vi "niDAQmx Timing (Implicit).vi"(0 "task in":refnum<class "Session Factory.lvclass">, 1 "samples per channel":i32=1000, 2 "sample mode":i32(ring)=10178 items=["Finite Samples"=10178, "Continuous Samples"=10123, "Hardware Timed Single Point"=12522], 11 "error in":errorcluster) -> (4 "task out":refnum<class "Session Factory.lvclass">, 15 "error out":errorcluster)   [LabVIEW 2021, in "Session Management niDAQmx.lvlib" / "Session Factory.lvclass"]
doc: "Sets only the number of samples to acquire or generate without specifying timing. Typically, you should use this instance when the task does not require sample timing, such as tasks that use counters for buffered frequency measurement, buffered period measurement, or pulse train generation. For finite counter output tasks, <B>samples per channel</B> is the number of pulses to generate."
uses:
  Session Factory.lvclass
  NI_DAQmx_client/RPC Messages/nidaqmx_grpc_CfgImplicitTimingRequest.ctl
  NI_DAQmx_client/RPC Messages/nidevice_grpc_Session.ctl
  NI_DAQmx_client/RPC Messages/nidevice_grpc_Session_session/nidevice_grpc_Session_session.lvclass
  NI_DAQmx_client/RPC Messages/nidaqmx_grpc_CfgImplicitTimingRequest_sample_mode_enum/nidaqmx_grpc_CfgImplicitTimingRequest_sample_mode_enum.lvclass
  Session Factory.lvclass/Session Factory.ctl
  NI_DAQmx_client/RPC Messages/nidaqmx_grpc_AcquisitionType.ctl
  NI_DAQmx_client/RPC Messages/nidaqmx_grpc_CfgImplicitTimingRequest_sample_mode_enum/nidaqmx_grpc_CfgImplicitTimingRequest_sample_mode_enum.lvclass/nidaqmx_grpc_CfgImplicitTimingRequest_sample_mode_enum.ctl
  NI_DAQmx_client/NI_DAQmx_client.lvlib
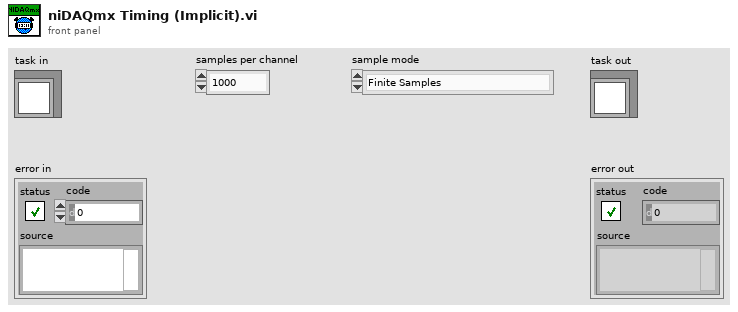
[diagram p1: front panel]
types:
  T1 = typedef "NI_DAQmx_client.lvlib/nidaqmx_grpc_CfgImplicitTimingRequest.ctl" = cluster{"task":T2, "nidaqmx_grpc_CfgImplicitTimingRequest_sample_mode_enum":refnum<class "nidaqmx_grpc_CfgImplicitTimingRequest_sample_mode_enum.lvclass">, "samps_per_chan":u64}
  T2 = typedef "NI_DAQmx_client.lvlib/nidevice_grpc_Session.ctl" = cluster{"nidevice_grpc_Session_session":refnum<class "nidevice_grpc_Session_session.lvclass">}
  T3 = typedef "NI_DAQmx_client.lvlib/nidaqmx_grpc_AcquisitionType.ctl" = enum32{"ACQUISITION_TYPE_UNSPECIFIED", "ACQUISITION_TYPE_FINITE_SAMPS", "ACQUISITION_TYPE_CONT_SAMPS", "ACQUISITION_TYPE_HW_TIMED_SINGLE_POINT"}
  T4 = typedef "grpc-lvsupport-release.lvlib/grpcId.ctl" = u64
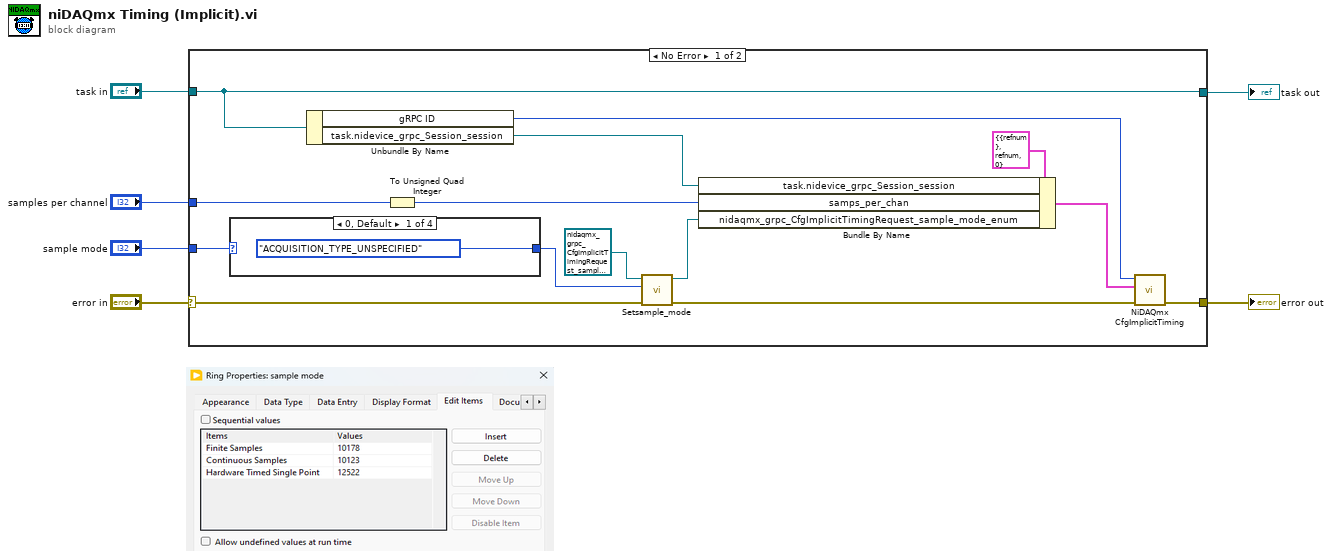
[diagram p0: block diagram]
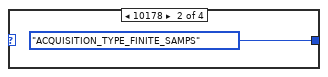
[diagram p2: hidden frame]
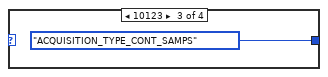
[diagram p3: hidden frame]
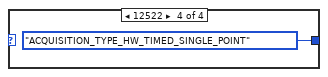
[diagram p4: hidden frame]
diagram:
  n1 = case shown="No Error" "error in" {
    selector: "error in" -> [w13 w26]
    tunnel: [w20 w26] -> w5
    tunnel: "task in" -> [w19 w25]
    tunnel: [w19 w25] -> w3
    tunnel: "samples per channel" -> [w9 _]
    tunnel: "sample mode" -> [w8 _]
    frame No Error {
      n2 = case shown="0, Default" w8 {
        tunnel: [nidaqmx_grpc_AcquisitionType."ACQUISITION_TYPE_UNSPECIFIED" ("Set_Val") nidaqmx_grpc_AcquisitionType."ACQUISITION_TYPE_FINITE_SAMPS" ("Set_Val") nidaqmx_grpc_AcquisitionType."ACQUISITION_TYPE_CONT_SAMPS" ("Set_Val") nidaqmx_grpc_AcquisitionType."ACQUISITION_TYPE_HW_TIMED_SINGLE_POINT" ("Set_Val")] -> w7
        frame 0, Default {
        }
        frame 10178 {
        }
        frame 10123 {
        }
        frame 12522 {
        }
      }
      n3 = Unbundle By Name(w19) -> ("gRPC ID"=w16:T4, "task.nidevice_grpc_Session_session"=w17:refnum<class "nidevice_grpc_Session_session.lvclass">)
      n4 = To Unsigned Quad Integer(1:w9) -> (0:w10:u64)
      n5 = call "Setsample_mode.vi"("error in (no error)"=w13, "Set_Val"=w7, "OneOfTemplate in"=refnum<class "nidaqmx_grpc_CfgImplicitTimingRequest_sample_mode_enum.lvclass"> refnum ("nidaqmx_grpc_CfgImplicitTimingRequest_sample_mode_enum")) -> ("error out"=w12:errorcluster, "OneOfTemplate out"=w11:refnum<class "nidaqmx_grpc_CfgImplicitTimingRequest_sample_mode_enum.lvclass">)  [unwired: 7 in]
      n6 = Bundle By Name(cluster=T1 {"task"={"nidevice_grpc_Session_session"=refnum}, "nidaqmx_grpc_CfgImplicitTimingRequest_sample_mode_enum"=refnum, "samps_per_chan"=0} ("Request Data"), "task.nidevice_grpc_Session_session"=w17, "samps_per_chan"=w10, "nidaqmx_grpc_CfgImplicitTimingRequest_sample_mode_enum"=w11) -> (w15:T1)
      n7 = call "NiDAQmx CfgImplicitTiming.vi"("error in"=w12, "Request Data"=w15, "gRPC ID"=w16) -> ("error out"=w20:errorcluster)  [unwired: 6 in, 2 out]
    }
    frame Error {
    }
  }
  "error out" <- w5
  "task out" <- w3
